vi "Phasor Find Intersections of Line Connecting References with Universal Circle.vi"(8 "Error In":errorcluster, 10 "Phasor 2":T1 {"s" format="%#_4g"; "g" format="%#_4g"}, 11 "Phasor 1":T1 {"s" format="%#_4g"; "g" format="%#_4g"}) -> (0 "Error Out":errorcluster, 1 "mu-":dbl format="%#_4g", 2 "Intersection 2":cluster{"x":dbl, "y":dbl} {"x" format="%#_4g"; "y" format="%#_4g"}, 3 "Intersection 1":cluster{"x":dbl, "y":dbl} {"x" format="%#_4g"; "y" format="%#_4g"}, 5 "mu+":dbl format="%#_4g")   [LabVIEW 2021, in "Phasor.lvlib"]
uses:
  Phasor (g, s).ctl
  <vilib>/Utility/error.llb/Error Cluster From Error Code.vi
  <vilib>/ErrorRing/Error Ring.xnode
  Phasor.lvlib
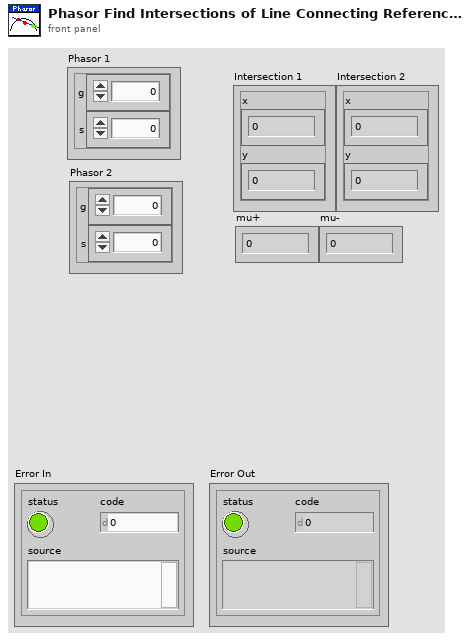
[diagram p1: front panel]
types:
  T1 = typedef "Phasor.lvlib/Phasor (g, s).ctl" = cluster{"g":dbl, "s":dbl}
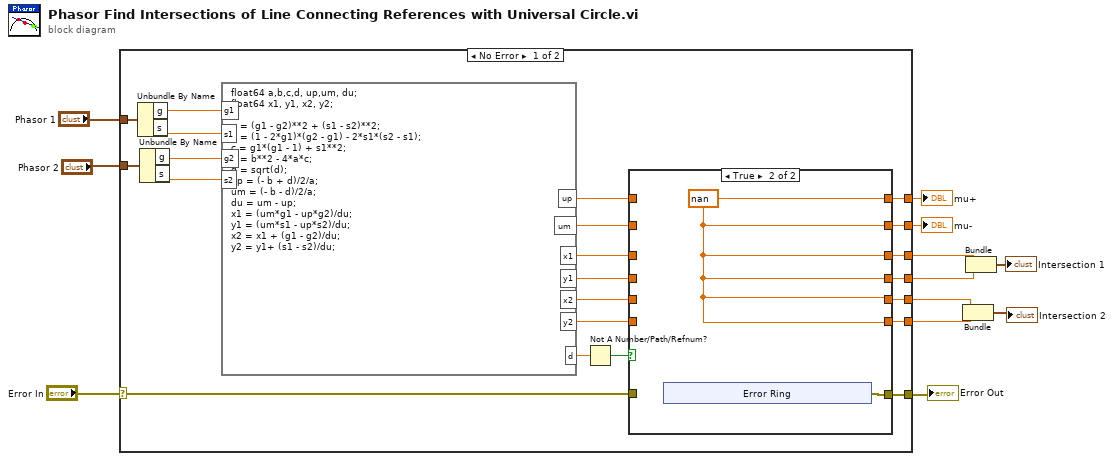
[diagram p0: block diagram]
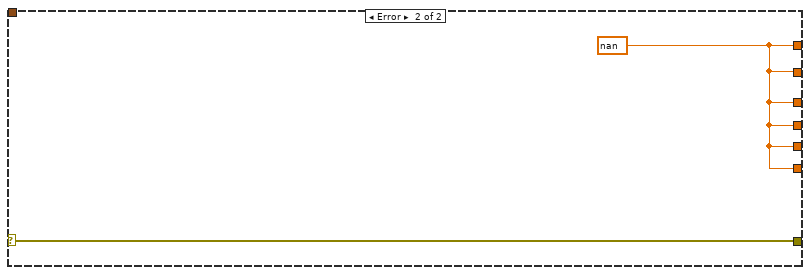
[diagram p3: hidden frame]
diagram:
  n1 = case shown="No Error" "Error In" {
    selector: "Error In" -> [w14 w49]
    tunnel: "Phasor 1" -> [w34 _]
    tunnel: "Phasor 2" -> [w31 _]
    tunnel: [w20 w48] -> w8
    tunnel: [w19 w48] -> w7
    tunnel: [w18 w48] -> w6
    tunnel: [w17 w48] -> w5
    tunnel: [w16 w48] -> w4
    tunnel: [w15 w48] -> w3
    tunnel: [w13 w49] -> w1
    frame No Error {
      n2 = Unbundle By Name(w34) -> ("g"=w33:dbl, "s"=w32:dbl)
      n3 = Unbundle By Name(w31) -> ("g"=w30:dbl, "s"=w29:dbl)
      n4 = formula code="float64 a,b,c,d, up,um, du;\nfloat64 x1, y1, x2, y2;\n\na = (g1 - g2)**2 + (s1 - s2)**2;\nb = (1 - 2*g1)*(g2 - g1) - 2*s1*(s2 - s1);\nc = g1*(g1 - 1) + s1**2;\nd = b**2 - 4*a*c;\nd = sqrt(d);\nup = (- b + d)/2/a;\num = (- b - d)/2/a;\ndu = um - up;\nx1 = (um*g1 - up*g2)/du;\ny1 = (um*s1 - up*s2)/du;\nx2 = x1 + (g1 - g2)/du;\ny2 = y1+ (s1 - s2)/du;"("s1"=w32, "s2"=w29, "g1"=w33, "g2"=w30) -> ("x1"=w24:dbl, "x2"=w22:dbl, "y1"=w23:dbl, "y2"=w21:dbl, "up"=w26:dbl, "um"=w25:dbl, "d"=w28:dbl)
      n5 = Not A Number/Path/Refnum?(number/path/refnum=w28) -> (NaN/Path/Refnum?=w27:bool)
      n6 = case shown="True" w27 {
        tunnel: w26 -> [w41 _]
        tunnel: w25 -> [w40 _]
        tunnel: w24 -> [w39 _]
        tunnel: w23 -> [w38 _]
        tunnel: w22 -> [w37 _]
        tunnel: w21 -> [w36 _]
        tunnel: [w41 w43] -> w20
        tunnel: [w40 w43] -> w19
        tunnel: [w39 w43] -> w18
        tunnel: [w38 w43] -> w17
        tunnel: [w37 w43] -> w16
        tunnel: [w36 w43] -> w15
        tunnel: w14 -> [w35 _]
        tunnel: [w35 w42] -> w13
        frame False {
        }
        frame True {
          w43 = nan
          n7 = xnode "Error Ring"() -> ("error out"=w42:errorcluster)
        }
      }
    }
    frame Error {
      w48 = nan
    }
  }
  "Error Out" <- w1
  "mu+" <- w8
  "mu-" <- w7
  n8 = Bundle(w4, w3) -> (→"Intersection 2":cluster{dbl, dbl})  [unwired: 1 in]
  n9 = Bundle(w6, w5) -> (→"Intersection 1":cluster{dbl, dbl})  [unwired: 1 in]
